vi "Keithley 622x Set Pulse Delta.vi"(4 "Width":dbl=0.0001 format="%#_6p", 5 "Average two pulses":bool, 6 "Step":dbl=0.0001 format="%#_6p", 7 "Delay":dbl=0.0001 format="%#_6p", 8 "error in":errorcluster, 9 "End":dbl=0.001 format="%#_6p", 10 "Start":dbl=-0.001 format="%#_6p", 11 "VISA resource name":refnum<visa-resource-name>) -> (0 "error out":errorcluster, 3 "VISA resource name out":refnum<visa-resource-name>)   [LabVIEW 2021]
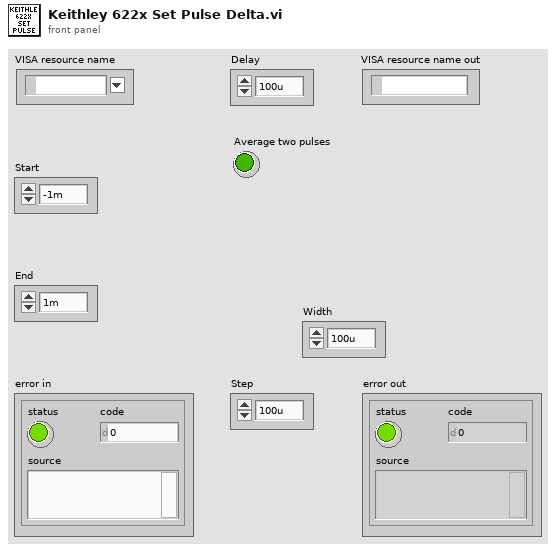
[diagram p1: front panel]
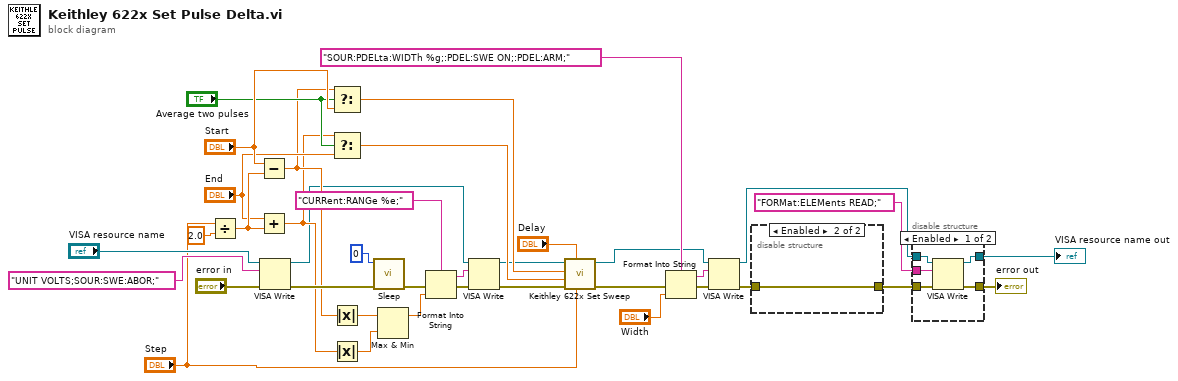
[diagram p0: block diagram]
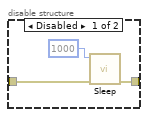
[diagram p3: hidden frame]
diagram:
  n1 = Divide(x="Step", y=2.0) -> (x/y=w17:dbl)
  n2 = Subtract(x="Start", y=w17) -> (x-y=w10:dbl)
  n3 = Add(x="End", y=w17) -> (x+y=w9:dbl)
  n4 = VISA Write(VISA resource name="VISA resource name", write buffer="UNIT VOLTS;SOUR:SWE:ABOR;", error in (no error)="error in") -> (VISA resource name out=w4:refnum<visa-resource-name>, error out=w24:errorcluster)  [unwired: 1 out]
  n5 = Select(t=w10, s="Average two pulses", f="Start") -> (s? t:f=w18:dbl)
  n6 = Select(t=w9, s="Average two pulses", f="End") -> (s? t:f=w14:dbl)
  n7 = Absolute Value(x=w10) -> (abs(x)=w11:dbl)
  n8 = Absolute Value(x=w9) -> (abs(x)=w12:dbl)
  n9 = call "Sleep.vi"("error in"=w24, "milliseconds to wait"=u32 0) -> ("error out"=w6:errorcluster)  [unwired: 9 in]
  n10 = Max & Min(x=w11, y=w12) -> (max(x,y)=w5:dbl)  [unwired: 1 out]
  n11 = Format Into String(format string="CURRent:RANGe %e;", error in=w6, w5) -> (resulting string=w7:string, error out=w2:errorcluster)  [unwired: 1 in]
  n12 = VISA Write(VISA resource name=w4, write buffer=w7, error in (no error)=w2) -> (VISA resource name out=w3:refnum<visa-resource-name>, error out=w1:errorcluster)  [unwired: 1 out]
  n13 = call "Keithley 622x Set Sweep.vi"("Step"="Step", "Delay"="Delay", "error in"=w1, "End"=w14, "Start"=w18, "VISA resource name"=w3) -> ("error out"=w26:errorcluster, "VISA resource name out"=w27:refnum<visa-resource-name>)  [unwired: 4 in]
  n14 = Format Into String(format string="SOUR:PDELta:WIDTh %g;:PDEL:SWE ON;:PDEL:ARM;", error in=w26, "Width") -> (resulting string=w37:string, error out=w38:errorcluster)  [unwired: 1 in]
  n15 = VISA Write(VISA resource name=w27, write buffer=w37, error in (no error)=w38) -> (VISA resource name out=w36:refnum<visa-resource-name>, error out=w34:errorcluster)  [unwired: 1 out]
  n16 = disable-structure shown="Enabled" {
    disable-tunnel: [w41 w42] -> w33
    disable-tunnel: w34 -> [w39 w42]
    frame Disabled {
      n17 = call "Sleep.vi"("error in"=w39, "milliseconds to wait"=u32 1000) -> ("error out"=w41:errorcluster)  [unwired: 9 in]
    }
    frame Enabled {
    }
  }
  n18 = disable-structure shown="Enabled" {
    disable-tunnel: w36 -> [w47 w48]
    disable-tunnel: "FORMat:ELEMents READ;" -> [w46 _]
    disable-tunnel: w33 -> [w45 w49]
    disable-tunnel: [w44 w49] -> w31
    disable-tunnel: [w43 w48] -> w30
    frame Enabled {
      n19 = VISA Write(VISA resource name=w47, write buffer=w46, error in (no error)=w45) -> (VISA resource name out=w43:refnum<visa-resource-name>, error out=w44:errorcluster)  [unwired: 1 out]
    }
    frame Disabled {
    }
  }
  "VISA resource name out" <- w30
  "error out" <- w31
